vi "Robot Global Data.vi"() -> ()   [LabVIEW 2017]
doc: "This global VI can contain as many global variables as you need. Place a control on the panel, give it a good name. To read or write to it from a VI, drag the icon to the diagram of that VI. You can also drag from the project. Click on the node to change which global you access. You shouldn't have multiple locations writing to a global or it will cause a race-condition."
uses:
  <vilib>/Rock Robotics/WPI/Camera/WPI_CameraImageSize.ctl
  <vilib>/Rock Robotics/WPI/DriverStation/WPI_DriverStationRobotMode2.ctl
  <vilib>/Rock Robotics/WPI/Solenoid/WPI_SolenoidValue.ctl
panel:
  out "Match Data":string
  out "Elbow Encoder":dbl
  out "AbsArm":dbl
  out "Tusk Right Encoder":dbl
  out "Tusk Left Encoder":dbl
  in  "State Arm":T1(ring)
  out "Solenoid Value":T2
  out "Auto Left Drive":dbl
  out "Auto Right Drive":dbl
  out "Joystick Y Axis":dbl
  out "Joystick X Axis":dbl
  out "TuskRight":dbl
  out "TuskLeft":dbl
  in  "Reset Encoder?":bool
  out "Angle":dbl
  out "EncoderValues":cluster{"EncoderLeft":dbl, "EncoderRight":dbl}
  in  "Reset Gyro?":bool
  in  "Robot Mode":T3
  in  "image size":T4=enum."320x240"
  in  "Enable Vision":bool
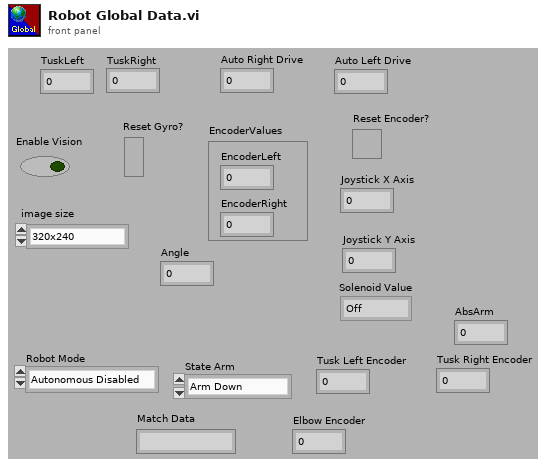
[diagram p1: front panel]
types:
  T1 = enum16{"Arm Down", "Arm Switch", "Arm(Low Scale)", "Arm(Normal Scale)", "Arm(High Scale)", "Hang"}
  T2 = typedef "WPI_SolenoidValue.ctl" = enum16{"Off", "On", "Forward", "Reverse"}
  T3 = typedef "WPI_DriverStationRobotMode2.ctl" = enum16{"Autonomous Disabled", "Autonomous Enabled", "Teleop Disabled", "Teleop Enabled", "Disconnected", "Finish", "Test Disabled", "Test Enabled", "Emergency Stopped"}
  T4 = typedef "WPI_CameraImageSize.ctl" = enum16{"640x480", "320x240", "160x120", "Custom"}
diagram:
